vi "Motor_ControllerPID.vi"(6 "Reinitialize? (F)":bool, 7 "PID Type (basic)":enum16{"basic", "adv"}(ring), 8 "error in (no error)":errorcluster, 10 "CableTensionRef(N)":dbl[](array[numeric]), 11 "Motor in":refnum<class "MotorControl.lvclass">) -> (0 "error out":errorcluster, 1 "PID cmd":dbl[](array[numeric]) format="%.2f", 2 "FF cmd":dbl[](array[numeric]), 3 "Motor out":refnum<class "MotorControl.lvclass">, 4 "FF+PID cmd":dbl[](array[numeric]), 5 "PID Gain Idx":i32[](array[numeric]))   [LabVIEW 2015, in "MotorControl.lvclass"]
uses:
  MotorControl.lvclass
  MotorControl.lvclass/MotorControl.ctl
  <vilib>/addons/control/pid/pid.llb/PID Advanced (DBL Array).vi
  <vilib>/addons/control/pid/pid.llb/PID Parameter Manager (DBL Array).vi
  <vilib>/addons/control/pid/pid.llb/PID Derivative Action Buffered (DBL Array).vi
  <vilib>/addons/control/pid/pid.llb/PID Get Advanced Error (DBL Array).vi
  <vilib>/addons/control/pid/pid.llb/PID Integral Action Buffered (DBL Array).vi
  <vilib>/addons/control/pid/pid.llb/PID Resize 1D Array.vi
  <vilib>/addons/control/pid/pid.llb/PID Get Advanced Error (DBL).vi
  <vilib>/addons/control/pid/pid.llb/PID Gain Schedule (DBL Array).vi
  <vilib>/addons/control/pid/pid.llb/PID (DBL Array).vi
  <vilib>/addons/control/pid/NI_PID_pid.lvlib
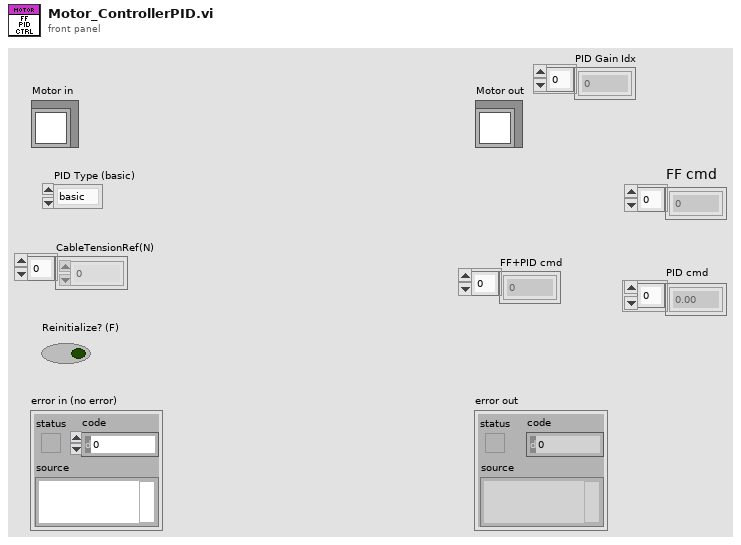
[diagram p1: front panel]
types:
  T1 = cluster{"setpoint high":dbl, "setpoint low":dbl}[]
  T2 = cluster{"PID gains":cluster{"proportional gain (Kc)":dbl, "integral time (Ti, min)":dbl, "derivative time (Td, min)":dbl}, "max value":dbl}[]
  T3 = cluster{"proportional gain (Kc)":dbl, "integral time (Ti, min)":dbl, "derivative time (Td, min)":dbl}[]
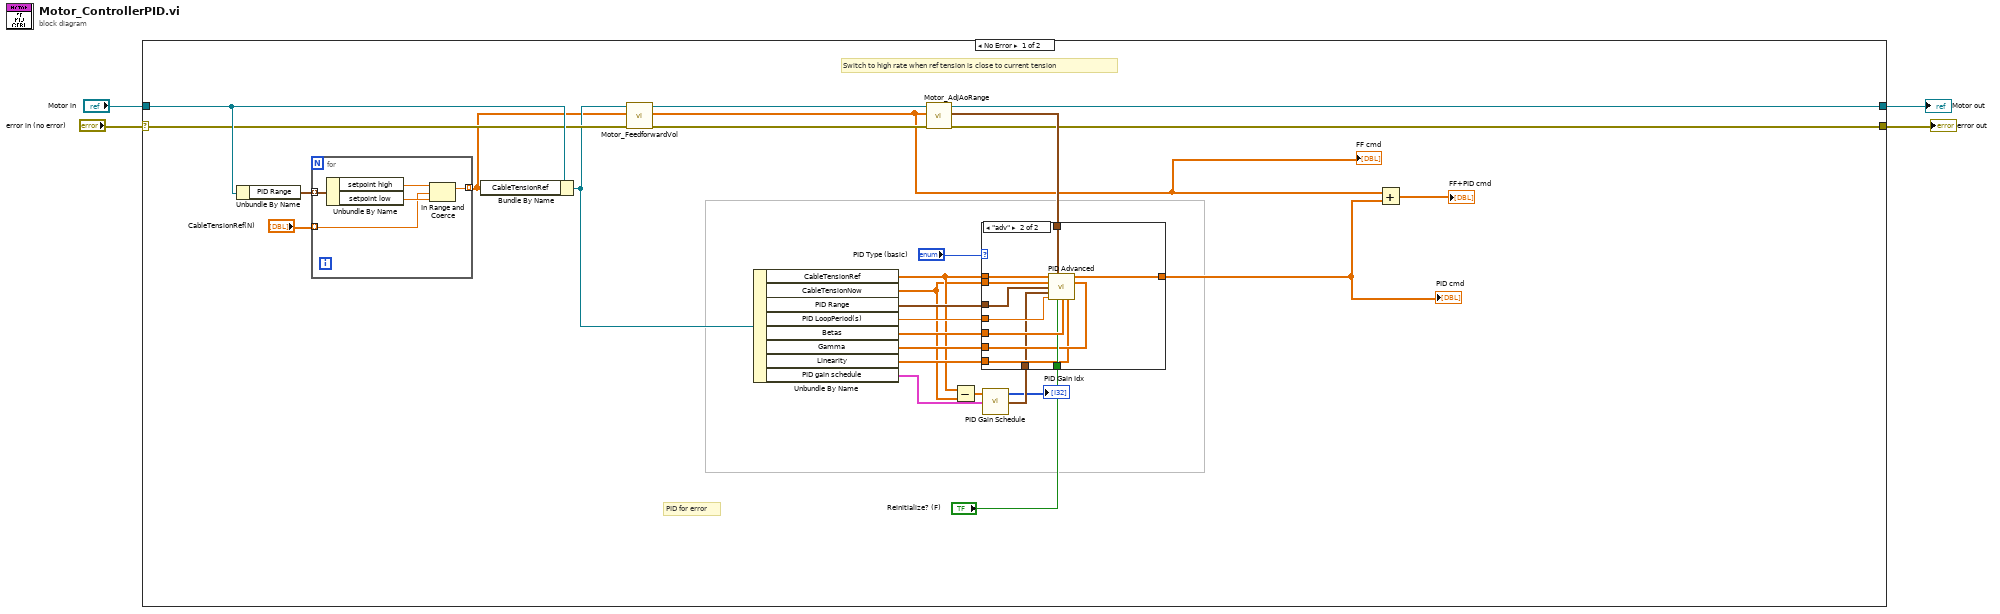
[diagram p0: block diagram]
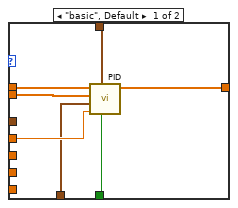
[diagram p2: hidden frame]
diagram:
  n1 = case shown="No Error" "error in (no error)" {
    selector: "error in (no error)" -> [w22 w56]
    tunnel: [w14 w56] -> w3
    tunnel: [w15 w55] -> w1
    tunnel: "Motor in" -> [w23 w55]
    frame No Error {
      # "Switch to high rate when ref tension is close to current tension"
      # "PID for error"
      n2 = Unbundle By Name(w23) -> ("PID Range"=w24:T1)
      n3 = for {
        tunnel: "CableTensionRef(N)" -> [w51] mode=indexing
        tunnel: w24 -> [w54] mode=indexing
        tunnel: [w50] -> w5 mode=indexing
        n4 = Unbundle By Name(w54) -> ("setpoint high"=w53:dbl, "setpoint low"=w52:dbl)
        n5 = In Range and Coerce(upper limit=w53, x=w51, lower limit=w52) -> (coerced(x)=w50:dbl)  [unwired: 1 out]
      }
      n6 = Bundle By Name(cluster=w23, "CableTensionRef"=w5) -> (w21:refnum<class "MotorControl.lvclass">)
      n7 = call "Motor_FeedforwardVol.vi"("error in (no error)"=w22, "TensionRef"=w5, "Motors_New in"=w21) -> ("error out"=w17:errorcluster, "FeedForwardVol"=w16:dbl[], "Motors_New out"=w18:refnum<class "MotorControl.lvclass">)  [unwired: 6 in]
      "FF cmd" <- w16
      n8 = Unbundle By Name(w21) -> ("CableTensionRef"=w9:dbl[], "CableTensionNow"=w8:dbl[], "PID Range"=w31:T1, "PID LoopPeriod(s)"=w30:dbl, "Betas"=w29:dbl[], "Gamma"=w20:dbl[], "Linearity"=w19:dbl[], "PID gain schedule"=w11:T2)
      n9 = call "Motor_AdjAoRange.vi"("error in (no error)"=w17, "FeedForwardVol"=w16, "Motors_New in"=w18) -> ("error out"=w14:errorcluster, "Adj AO Range"=w27:cluster{"output high":dbl, "output low":dbl}[], "Motors_New out"=w15:refnum<class "MotorControl.lvclass">)  [unwired: 6 in]
      n10 = Subtract(x=w9, y=w8) -> (x-y=w10:dbl[])
      n11 = call-poly <vilib>:"PID Gain Schedule.vi"("PID gain schedule"=w11, "gain scheduling value"=w10) -> ("PID gains out"=w12:T3, "index out"=→"PID Gain Idx":i32[])  [unwired: 2 in]
      n12 = case shown="\"adv\"" "PID Type (basic)" {
        tunnel: w31 -> [_ w49]
        tunnel: w30 -> [w33 w48]
        tunnel: w29 -> [_ w47]
        tunnel: "Reinitialize? (F)" -> [w34 w46]
        tunnel: w27 -> [w38 w45]
        tunnel: w20 -> [_ w44]
        tunnel: w19 -> [_ w43]
        tunnel: [w35 w42] -> w13
        tunnel: w12 -> [w32 w41]
        tunnel: w9 -> [w37 w40]
        tunnel: w8 -> [w36 w39]
        frame "basic", Default {
          n13 = call-poly <vilib>:"PID.vi"("reinitialize? (F)"=w34, "output range"=w38, "dt (s)"=w33, "PID gains"=w32, "process variable"=w36, "setpoint"=w37) -> ("output"=w35:dbl[])  [unwired: 4 in, 1 out]
        }
        frame "adv" {
          n14 = call-poly <vilib>:"PID Advanced.vi"("setpoint"=w40, "output range"=w45, "process variable"=w39, "gamma"=w44, "setpoint range"=w49, "PID gains"=w41, "dt (s)"=w48, "reinitialize? (F)"=w46, "beta"=w47, "linearity"=w43) -> ("output"=w42:dbl[])  [unwired: 4 in, 1 out]
        }
      }
      "PID cmd" <- w13
      n15 = Add(x=w16, y=w13) -> (x+y=→"FF+PID cmd":dbl[])
    }
    frame Error {
    }
  }
  "error out" <- w3
  "Motor out" <- w1
